vi "CurrentInputDelete.vi"(8 "error in":errorcluster, 11 "Device In":u64) -> (0 "error out":errorcluster)   [LabVIEW 2020, in "Phidget Current Input.lvlib"]
doc: "Deletes a Phidget Current Input"
uses:
  <instrlib>/Phidgets/Phidget Current Input/Phidget Current Input.lvlib
  <instrlib>/Phidgets/Phidget Common/Phidget Common.lvlib
  phidget22.dll
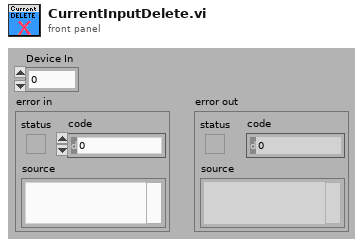
[diagram p1: front panel]
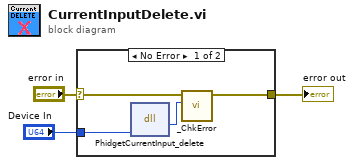
[diagram p0: block diagram]
diagram:
  n1 = case shown="No Error" "error in" {
    selector: "error in" -> [w5 w8]
    tunnel: [w4 w8] -> w2
    tunnel: "Device In" -> [w6 _]
    frame No Error {
      n2 = dll-call lib="phidget22.*" fn="PhidgetCurrentInput_delete"("phid"=w6) -> ("return type"=w7:i32)  [unwired: 4 in, 2 out]
      n3 = call <instrlib>:"_ChkError.vi"("Return Code"=w7, "error in (no error)"=w5) -> ("error out"=w4:errorcluster)  [unwired: 9 in]
    }
    frame Error {
    }
  }
  "error out" <- w2
